vi "DecodeStringList.vi"(8 "error in (no error)":errorcluster, 11 "String List (\"<STR1>\",\"<STR2>\",...)":string) -> (0 "error out":errorcluster, 3 "String as Array":string[](array[string]))   [LabVIEW 2018, in "OXYGEN.lvlib"]
uses:
  OXYGEN.lvlib
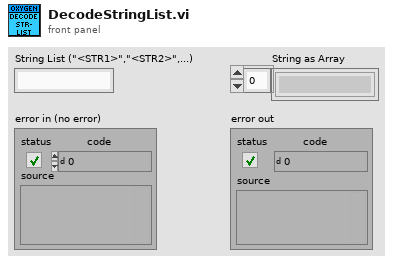
[diagram p1: front panel]
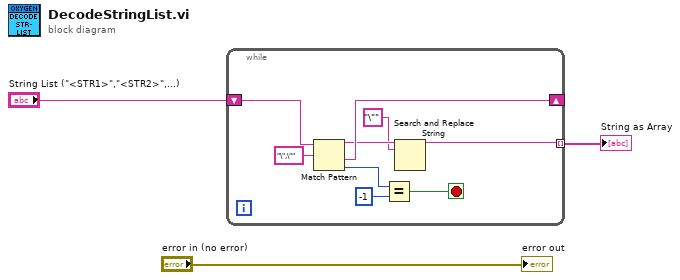
[diagram p0: block diagram]
diagram:
  n1 = while {
    shift-right: [w7] -> _
    shift-left: "String List (\"<STR1>\",\"<STR2>\",...)" -> [w9]
    tunnel: [w4] -> w2 mode=indexing
    stop <- w10 stop-if-true
    n2 = Match Pattern(string=w9, regular expression="\",\"") -> (before substring=w6:string, after substring=w7:string, offset past match=w12:i32)  [unwired: 1 in, 1 out]
    n3 = Equal?(x=w12, y=-1) -> (x = y?=w10:bool)
    n4 = Search and Replace String(input string=w6, search string="\"" ("substring (\"\")")) -> (result string=w4:string)  [unwired: 6 in, 3 out]
  }
  "String as Array" <- w2
  "error out" <- "error in (no error)"
